vi "DataLogging (SubVI).vi"(8 "error in (no error)":errorcluster, 10 "data to file":dbl[](array[numeric]), 11 "Refnum in":refnum<k34>) -> (0 "error out":errorcluster, 3 "Refnum out":refnum<k34>)   [LabVIEW 2018]
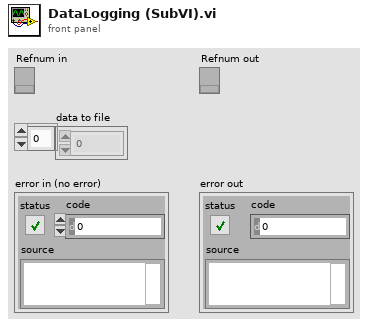
[diagram p1: front panel]
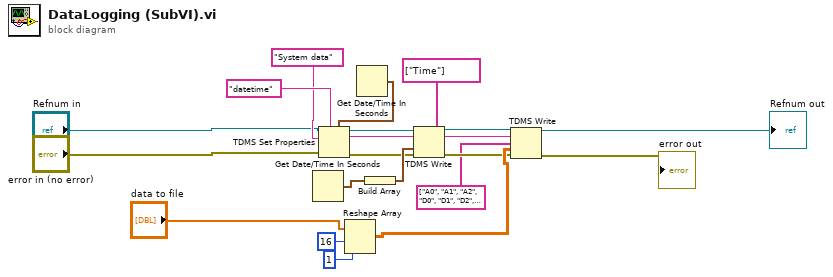
[diagram p0: block diagram]
diagram:
  n1 = Get Date/Time In Seconds() -> (seconds since 1Jan1904=w17:timestamp)
  n2 = Reshape Array("data to file", 16 ("dimension size"), 1 ("dimension size")) -> (w21:dbl[][])
  n3 = Get Date/Time In Seconds() -> (seconds since 1Jan1904=w10:timestamp)
  n4 = TDMS Set Properties(5:w10, 7:"datetime", 8:"error in (no error)", 10:"System data" ("group name in (Untitled)"), 11:"Refnum in") -> (0:w12:errorcluster, 2:w15:string, 3:w11:refnum<k34>)  [unwired: 1 in, 1 out]
  n5 = Build Array(w17) -> (w18:timestamp[])
  n6 = TDMS Write(0:w11, 5:w15, 7:string[] ["Time"] ("channel name(s) in (Untitled)"), 9:w18, 11:w12) -> (4:w13:refnum<k34>, 6:w16:string, 15:w14:errorcluster)  [unwired: 1 in, 1 out]
  n7 = TDMS Write(0:w13, 5:w16, 7:string[] ["A0", "A1", "A2", "D0", "D1", "D2", "T0", "CA0", "TJ0", "F", "F0", "Fj", "L", "CA", "T", "TJ"] ("channel name(s) in (Untitled)"), 9:w21, 11:w14) -> (4:→"Refnum out":refnum<k34>, 15:→"error out":errorcluster)  [unwired: 1 in, 2 out]
